vi "Proceed.vi"(7 "component is ready (Y)":bool=TRUE, 8 "error in (no error)":errorcluster, 10 "ProceedMessage":refnum<class "ProceedMessage.lvclass">, 11 "Trace in":refnum<class "Trace.lvclass">) -> (0 "error out":errorcluster, 2 "all observers are ready?":bool, 3 "Trace out":refnum<class "Trace.lvclass">)   [LabVIEW 2012, in "Trace.lvclass"]
doc: "The Proceed method is used to check if your component is ready. Also it checks if the observers are ready. When the observers and the component are ready, it sends the proceed to its observee. If it's the highest observee, it distributes a stop command."
uses:
  Trace.lvclass
  <vilib>/Distrio/Murmex/Murmex/Murmex.lvclass
  <vilib>/Distrio/Murmex/ProceedMessage/ProceedMessage.lvclass
panel:
  # "This method is called when the PROCEED\ntrigger is sent. \n\nOverride this method when your component needs to\nrespond to this trigger. \n\nCall parent for proper implementation"
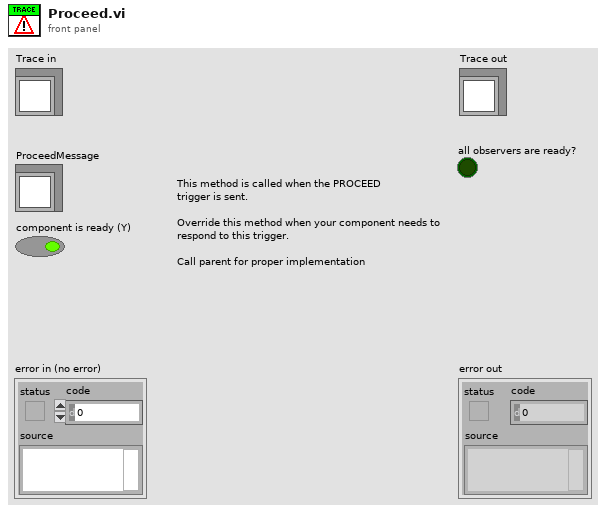
[diagram p1: front panel]
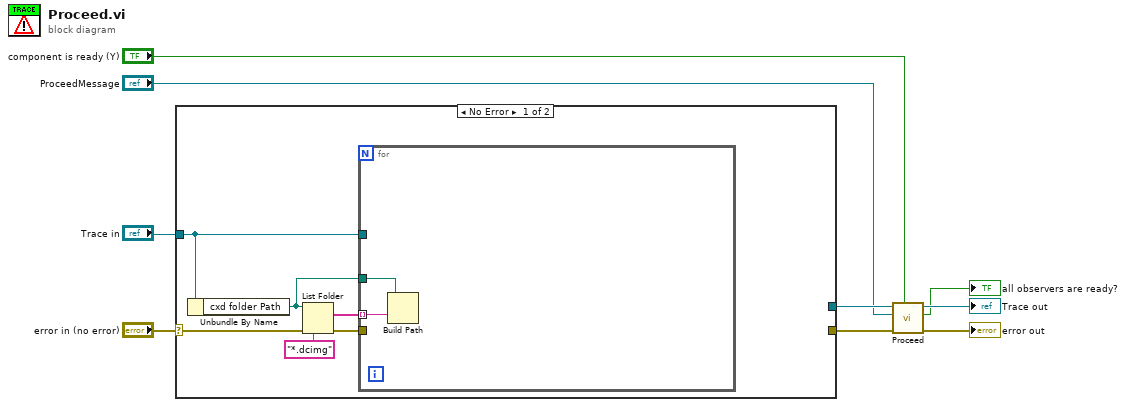
[diagram p0: block diagram]
diagram:
  n1 = case shown="No Error" "error in (no error)" {
    selector: "error in (no error)" -> [w15 w19]
    tunnel: "Trace in" -> [w11 w18]
    tunnel: [_ w19] -> w6
    tunnel: [_ w18] -> w4
    frame No Error {
      n2 = Unbundle By Name(w11) -> ("cxd folder Path"=w10:path)
      n3 = List Folder(path=w10, pattern="*.dcimg", error in=w15) -> (filenames=w12:string[], error out=w13:errorcluster)  [unwired: 1 in, 2 out]
      n4 = for {
        tunnel: w13 -> [_]
        tunnel: w12 -> [w17] mode=indexing
        tunnel: w11 -> [_]
        tunnel: w10 -> [w16]
        n5 = Build Path(base path=w16, name or relative path=w17) -> ()  [unwired: 1 out]
      }
    }
    frame Error {
    }
  }
  n6 = call-parent "Proceed.vi"("component is ready (Y)"="component is ready (Y)", "error in (no error)"=w6, "ProceedMessage"="ProceedMessage", "Murmex in"=w4) -> ("error out"=→"error out":errorcluster, "all observers are ready?"=→"all observers are ready?":bool, "Murmex out"=→"Trace out":refnum<class "Trace.lvclass">)  [unwired: 5 in]
